vi "JOG.vi"(0 "System no.":i32=1 min=1 max=4 step=1, 2 "Axes to jog":string[](array[string]), 3 "JOG velocity":dbl[](array[numeric]) format="%.6f", 4 "No.of digits":i16=4, 5 "error in":errorcluster) -> (19 "error out":errorcluster)   [LabVIEW 2020]
doc: "Starts motion with the given (constant) velocity values for the specified axes. The sign of the velocity values determines the direction of motion.\nWhen motion started with JOG is executed, the target value is changed continuously according to the given velocity (can be checked with MOV?.vi). \nMotion started with JOG is executed in addition to motion started with other move commands (e.g. MOV.vi or MVR.vi ).\nAs long as motion of the axis is caused by JOG only, the axis stays on target (i.e. ONT?.vi responds with 1 since the target is continuously adapted to the actual motion). \nMotion started by JOG is stopped in the following cases:\n- The velocity is set to 0 with JOG.\n- #24, STP or HLT is sent: these commands set the velocity for JOG to 0.\n- A travel range limit is reached: the velocity for JOG remains unchanged, no error is set, the target value is set equal to the limit value.\nJOG can be changed while the axis is moving."
panel:
  # "Starts motion with the given (constant) velocity for the given axis."
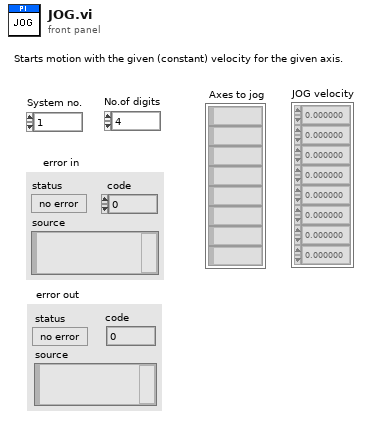
[diagram p1: front panel]
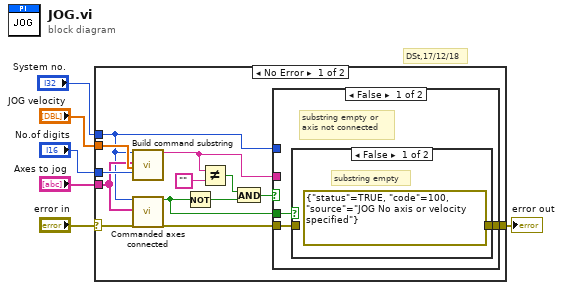
[diagram p0: block diagram]
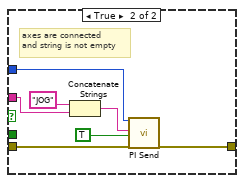
[diagram p3: hidden frame]
diagram:
  # "DSt,17/12/18"
  n1 = case shown="No Error" "error in" {
    selector: "error in" -> [w7 w32]
    tunnel: [w19 w32] -> w6
    tunnel: "JOG velocity" -> [w16 _]
    tunnel: "No.of digits" -> [w15 _]
    tunnel: "System no." -> [w8 _]
    tunnel: "Axes to jog" -> [w13 _]
    frame No Error {
      n2 = call "Build command substring.vi"("System no."=w8, "Affected axes"=w13, "Parameters"=w16, "No. of digits"=w15) -> ("Command substring"=w17:string)  [unwired: 3 in, 12 out]
      n3 = call "Commanded axes connected.vi"("System no."=w8, "Commanded axes"=w13, "error in"=w7) -> ("Controller error"=w11:bool, "error out"=w14:errorcluster)  [unwired: 1 in, 14 out]
      n4 = Not(x=w11) -> (.not. x?=w10:bool)
      n5 = Not Equal?(x=w17, y="") -> (x != y?=w12:bool)
      n6 = And(x=w12, y=w10) -> (x .and. y?=w9:bool)
      n7 = case shown="False" w9 {
        tunnel: w17 -> [_ w30]
        tunnel: [w22 w26] -> w19
        tunnel: w14 -> [w20 w27]
        tunnel: w11 -> [w21 _]
        tunnel: w8 -> [_ w25]
        frame False {
          # "substring empty or \naxis not connected"
          n8 = case shown="False" w21 {
            tunnel: [errorcluster {"status"=TRUE, "code"=100, "source"="JOG No axis or velocity specified"} ("error out") w24] -> w22
            tunnel: w20 -> [_ w24]
            frame False {
              # "substring empty"
            }
            frame True {
              # "commanded axis\nnot connected"
            }
          }
        }
        frame True {
          # "axes are connected \nand string is not empty"
          n9 = Concatenate Strings("JOG", w30) -> (w28:string)
          n10 = call "PI Send.vi"("System no."=w25, "String to send"=w28, "Attach termination char.?"=TRUE ("Attach Linefeed?"), "error in"=w27) -> ("error out"=w26:errorcluster)  [unwired: 2 in, 13 out]
        }
      }
    }
    frame Error {
    }
  }
  "error out" <- w6
